vi "SpinUp.vi"(11 "Button":bool) -> ()   [LabVIEW 2016]
uses:
  <vilib>/Rock Robotics/WPI/ThirdParty/CanMotor/TalonSRX/WPI_CANTalonSRX_APIControlMode.ctl
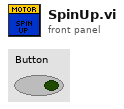
[diagram p1: front panel]
types:
  T1 = typedef "WPI_CANTalonSRX_APIControlMode.ctl" = enum8{"Percent VBus", "Speed", "Position", "Slave", "Unchanged / Invalid", "Voltage Compensation", "Current", "Motion Profile", "Motion Magic"}
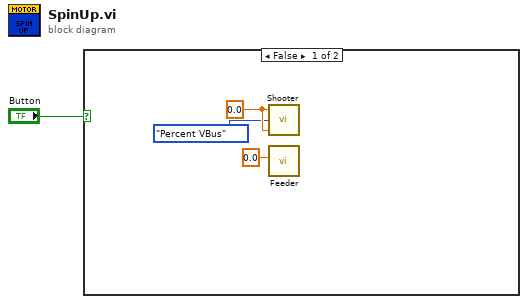
[diagram p0: block diagram]
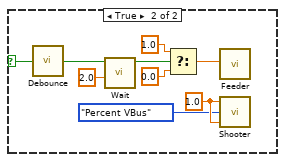
[diagram p2: hidden frame]
diagram:
  n1 = case shown="False" "Button" {
    selector: "Button" -> [_ w8]
    frame False {
      w3 = 0.0 ("Power")
      n2 = call "Shooter.vi"("FrontMotorIn"=w3, "Control Mode"=WPI_CANTalonSRX_APIControlMode."Percent VBus", "RearMotorIn"=w3) -> ()  [unwired: 1 in]
      n3 = call "Feeder.vi"("Power"=0.0) -> ()  [unwired: 11 in]
    }
    frame True {
      w6 = 1.0 ("Power")
      n4 = call "Debounce.vi"("Input"=w8) -> ("Output"=w7:bool)
      n5 = call "Wait.vi"("Target Time (s)"=2.0 ("Target Time"), "First Time?"=w7) -> ("Completed"=w12:bool)  [unwired: 9 in]
      n6 = Select(t=1.0, s=w12, f=0.0) -> (s? t:f=w9:dbl)
      n7 = call "Feeder.vi"("Power"=w9) -> ()  [unwired: 11 in]
      n8 = call "Shooter.vi"("FrontMotorIn"=w6, "Control Mode"=WPI_CANTalonSRX_APIControlMode."Percent VBus", "RearMotorIn"=w6) -> ()  [unwired: 1 in]
    }
  }
